vi "Graph Scale Maker.vi"(8 "Logarithm?":bool, 9 "Value Pair Info Array":cluster{"Value":sgl, "Name":string}[](array[cluster]), 10 "Major Ticks":u16, 11 "Range In":cluster{"Max":sgl, "Min":sgl}) -> (1 "Maker Array":sgl[](array[numeric]), 2 "Mapping Mode":u8, 3 "Range Out":cluster{"Max":sgl, "Min":sgl})   [LabVIEW 2017, in "3D Plot.lvclass"]
uses:
  <vilib>/Math Plots/3D Math Plots/3D Plot/3D Plot/3D Plot.lvclass
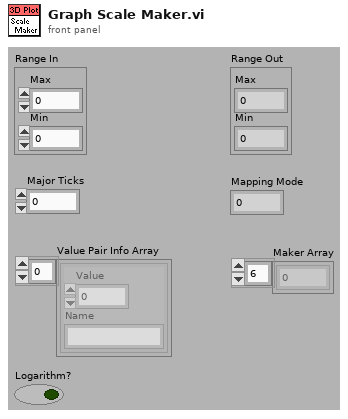
[diagram p1: front panel]
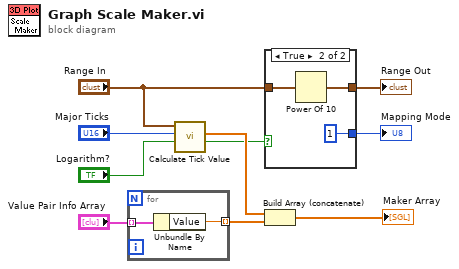
[diagram p0: block diagram]
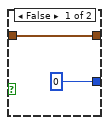
[diagram p2: hidden frame]
diagram:
  n1 = for {
    tunnel: "Value Pair Info Array" -> [w12] mode=indexing
    tunnel: [w11] -> w10 mode=indexing
    n2 = Unbundle By Name(w12) -> ("Value"=w11:sgl)
  }
  n3 = call <vilib>:"Calculate Tick Value.vi"("Logarithm?"="Logarithm?", "Tick Count"="Major Ticks", "Axis Range"="Range In") -> ("Logarithm?"=w4:bool, "Tick Value Array"=w8:sgl[])  [unwired: 1 in, 6 out]
  n4 = case shown="True" w4 {
    tunnel: [u8 0 u8 1] -> w3
    tunnel: "Range In" -> [w14 w16]
    tunnel: [w14 w15] -> w1
    frame False {
    }
    frame True {
      n5 = Power Of 10(x=w16) -> (10^x=w15:cluster{"Max":sgl, "Min":sgl})
    }
  }
  "Mapping Mode" <- w3
  "Range Out" <- w1
  n6 = Build Array (concatenate)(w8, w10) -> (→"Maker Array":sgl[])
